vi "BLE_Notify.vi"(0 ".NET Refnum in":refnum<k24>, 5 "UUID":string, 7 "WriteByteArray":u8[](array[numeric]), 11 "error in (no error)":errorcluster) -> (4 ".NET Refnum out":refnum<k24>, 10 "Result":string, 15 "error out":errorcluster)   [LabVIEW 2020, in "BLE.lvlib"]
uses:
  C:/Users/Trait/Desktop/LabView Project/LabView BLE DataACQ/BLELib.dll
  BLELib.dll
  BLE.lvlib
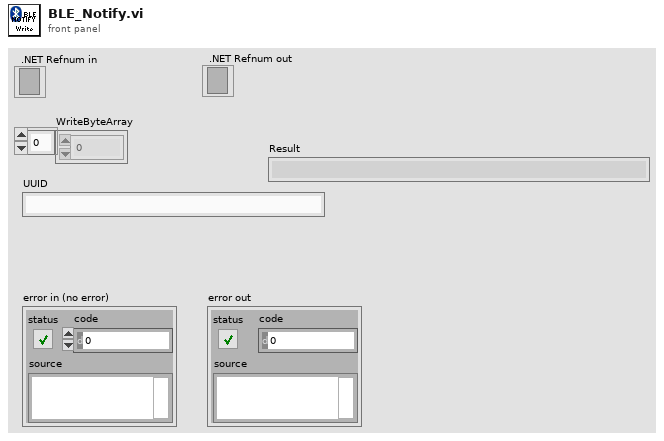
[diagram p1: front panel]
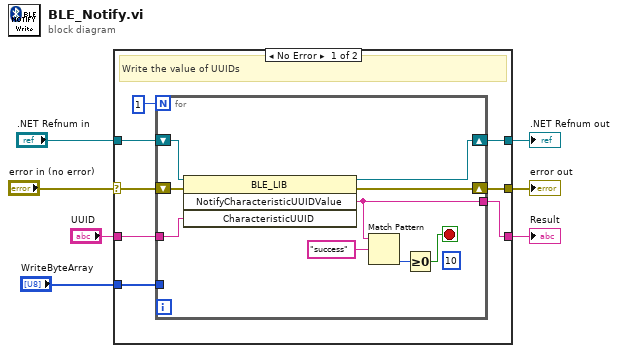
[diagram p0: block diagram]
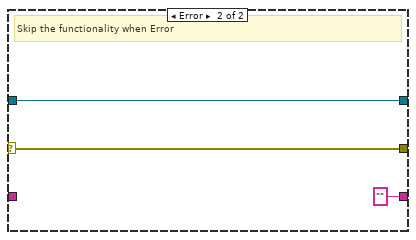
[diagram p2: hidden frame]
diagram:
  n1 = case shown="No Error" "error in (no error)" {
    selector: "error in (no error)" -> [w12 w27]
    tunnel: "UUID" -> [w15 _]
    tunnel: "WriteByteArray" -> [w14 _]
    tunnel: [w13 "" ("Result")] -> w5
    tunnel: [w11 w27] -> w3
    tunnel: [w10 w26] -> w2
    tunnel: ".NET Refnum in" -> [w9 w26]
    frame No Error {
      # "Write the value of UUIDs"
      n2 = for {
        N: 1 -> [_]
        tunnel: w15 -> [w18]
        tunnel: w14 -> [_]
        tunnel: [w17] -> w13
        shift-right: [w16] -> w11
        shift-left: w12 -> [w24]
        shift-right: [w23] -> w10
        shift-left: w9 -> [w19]
        stop <- w20 stop-if-true
        (unwired) 10
        n3 = invoke class="BLE_LIB" method="NotifyCharacteristicUUIDValue"(reference=w19, error in=w24, "CharacteristicUUID"=w18) -> (reference out=w23:refnum<k24>, error out=w16:errorcluster, "NotifyCharacteristicUUIDValue"=w17:string)  [unwired: 1 in, 1 out]
        n4 = Match Pattern(string=w17, regular expression="success") -> (offset past match=w21:i32)  [unwired: 1 in, 3 out]
        n5 = Greater Or Equal To 0?(x=w21) -> (x >= 0?=w20:bool)
      }
    }
    frame Error {
      # "Skip the functionality when Error"
    }
  }
  "Result" <- w5
  "error out" <- w3
  ".NET Refnum out" <- w2
